vi "Do.vi"(8 "error in (no error)":errorcluster, 10 "Actor in":refnum<class "Actor.lvclass">, 11 "scan2d_perform_scan Msg":refnum<class "scan2d_perform_scan Msg.lvclass">) -> (0 "error out":errorcluster, 2 "Actor out":refnum<class "Actor.lvclass">)   [LabVIEW 2015, in "scan2d_perform_scan Msg.lvclass"]
doc: "This VI delivers the message to the actor by calling the appropriate method(s) on the actor."
uses:
  scan2d_perform_scan Msg.lvclass
  <vilib>/ActorFramework/Actor/Actor.lvclass
  2d_scan/scan_2d.lvclass
  scan2d_perform_scan Msg.lvclass/scan2d_perform_scan Msg.ctl
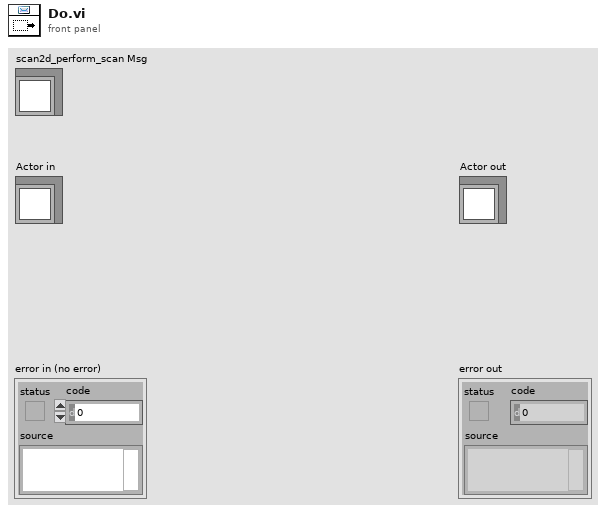
[diagram p1: front panel]
types:
  T1 = typedef "scan_2d_settings.ctl" = cluster{"X Start":dbl, "X Stop":dbl, "X Steps":u32, "Y Start":dbl, "Y Stop":dbl, "Y Steps":u32, "Integration Time":dbl, "Record Type":T2, "Save Path":path, "Stage Number":enum16{"1", "2"}, "notes":string}
  T2 = typedef "scan_record.ctl" = enum16{"hdf5", "legacy", "None"}
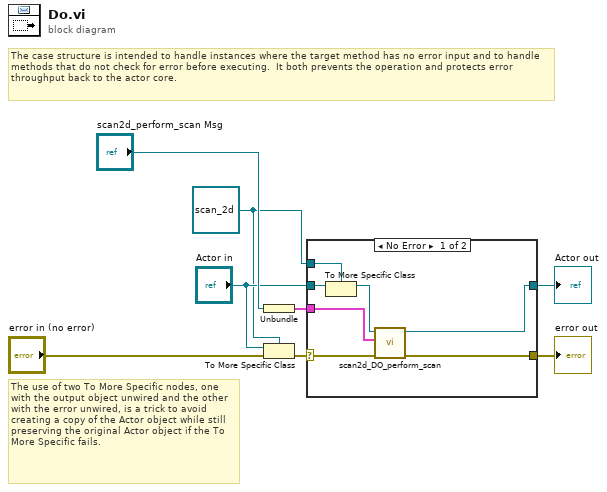
[diagram p0: block diagram]
diagram:
  w2 = refnum<class "scan_2d.lvclass"> refnum ("Actor in")
  # "The use of two To More Specific nodes, one with the output object unwired and the other with the error unwired, is a trick to avoid creating a copy of the Actor object while still preserving the original Actor object if the To More Specific fails."
  # "The case structure is intended to handle instances where the target method has no error input and to handle methods that do not check for error before executing.  It both prevents the operation and protects error throughput back to the actor core."
  n1 = Unbundle("scan2d_perform_scan Msg") -> (w1:T1)
  n2 = To More Specific Class(target class=w2, reference="Actor in", error in="error in (no error)") -> (error out=w6:errorcluster)  [unwired: 1 out]
  n3 = case shown="No Error" w6 {
    selector: w6 -> [w13 w17]
    tunnel: [w15 w17] -> w5
    tunnel: [w14 w16] -> w4
    tunnel: "Actor in" -> [w12 w16]
    tunnel: w2 -> [w11 _]
    tunnel: w1 -> [w9 _]
    frame No Error {
      n4 = To More Specific Class(target class=w11, reference=w12) -> (specific class reference=w10:refnum<class "scan_2d.lvclass">)  [unwired: 1 in, 1 out]
      n5 = call "scan2d_DO_perform_scan.vi"("error in (no error)"=w13, "scan-2d-settings"=w9, "scan_panel in"=w10) -> ("error out"=w15:errorcluster, "scan_panel out"=w14:refnum<class "scan_2d.lvclass">)  [unwired: 7 in]
    }
    frame Error {
      # "If type check fails, pass the original object out again."
    }
  }
  "error out" <- w5
  "Actor out" <- w4
